vi "Create Value - Array.vi"(8 "error in (no error)":errorcluster) -> (0 "error out":errorcluster, 3 "JSON Tree":variant)   [LabVIEW 2014, in "i3-json.lvlib"]
doc: "Creates a new JSON Object of the given type"
uses:
  i3-json.lvlib
  JSON Types/JSON Type.ctl
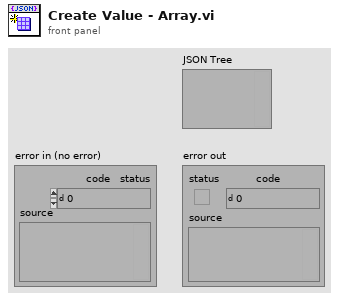
[diagram p1: front panel]
types:
  T1 = typedef "i3-json.lvlib/JSON Type.ctl" = enum8{"JSON Compatible", "JSON Array", "JSON Object", "JSON Null", "Double", "String", "Boolean", "Unknown"}
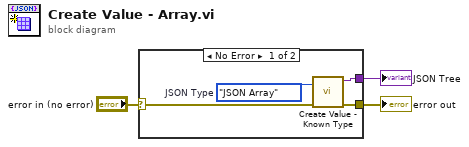
[diagram p0: block diagram]
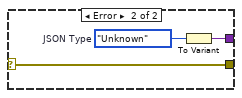
[diagram p2: hidden frame]
diagram:
  n1 = case shown="No Error" "error in (no error)" {
    selector: "error in (no error)" -> [w4 w8]
    tunnel: [w5 w8] -> w2
    tunnel: [w6 w9] -> w1
    frame No Error {
      w7 = JSON_Type."JSON Array"  # JSON Type
      n2 = call "Create Value - Known Type.vi"("JSON Type"=w7, "error in (no error)"=w4) -> ("error out"=w5:errorcluster, "JSON Tree"=w6:variant)  [unwired: 8 in]
    }
    frame Error {
      w10 = JSON_Type."Unknown"  # JSON Type
      n3 = To Variant(anything=w10) -> (Variant=w9:variant)
    }
  }
  "JSON Tree" <- w1
  "error out" <- w2
